vi "Sweep control.vi"(0 "Scan control":cluster{"Priority":u16, "Scan name":u16}[](array[cluster])=[{"Priority"=0, "Scan name"=1}, {"Priority"=1, "Scan name"=5}, {"Priority"=3, "Scan name"=0}, {"Priority"=2, "Scan name"=0}] {"Scan name" items=["OFF", "Vsg1", "Vsg2", "Vsgw", "Vbg", "Field", "Temp", "MW_freq", "MW_amplitude"]; "Priority" items=["Priority 0", "Priority 1", "Priority 2", "Priority 3", "Priority 4", "Priority 5"]}, 1 "Scan parameters":T2(array[cluster])=[{"DAQ Channel"=3, "Label"="\nappliedVsg=", "Scaled low"=-0.1, "Scaled high"=0.6, "Start"=-0.015, "End"=0.2, "Step"=0.001, "Scale?"=FALSE, "Output-Not Used"=0}, {"DAQ Channel"=3, "Label"="\nappliedField=", "Scaled low"=-0.175, "Scaled high"=0.775, "Start"=5.0, "End"=3.0, "Step"=0.1, "Scale?"=FALSE, "Output-Not Used"=2}, {"DAQ Channel"=3, "Label"="\nappliedVbg=", "Scaled low"=-0.11, "Scaled high"=0.31, "Start"=-1.55, "End"=3.0, "Step"=0.015, "Scale?"=FALSE, "Output-Not Used"=2}, {"DAQ Channel"=3, "Label"="\nappliedField=", "Scaled low"=-0.060000000000000005, "Scaled high"=0.14, "Start"=0.0, "End"=10000.0, "Step"=5000.0, "Scale?"=FALSE, "Output-Not Used"=2}] {"Step" format="%#_6p"; "End" format="%#_6p"; "Start" format="%#_6p"; "Scaled high" format="%#_6p"; "Scaled low" format="%#_6p"}, 3 "Comments":string="SA02703M.20141208\nVbg=0.25VV\n\nB= +0T\nSweep Vsg: -115mV to 200mV, 1mV steps\n\nlockin\n0: 1, current 2.5mV AC 400uV DC, 400mHz\n1: 2\n2: 3\n3: 5, \n4: 7, current\n5: 9, ", 4 "Experiment folder name":string="1 - seep Vsg") -> ()   [LabVIEW 2013]
uses:
  <userlib>/Levylab/DAQ-Lockin-SubVI/Lockin-4461_MultiChannel - IV 3.0 globals.vi
  Labview_Local/Lockin-4461_Multiple Inputs and Outputs_KH Folder/P/users1/Joe/Lockin-4461_3.0 4461-4462 Multichannel Folder/DAQ-Lockin-SubVI/Lock-in Globles Multiple Inputs and Outputs.vi
panel:
  in  "Channels: AO":T1={"AO amp (V)"=[0.002, 0.002, 0.002, 0.002, 0.002, 0.002, 0.002, 0.002], "AO DC (V)"=[0.0, 0.0, 0.0, 0.0, 0.0, 0.0, 0.0, 0.0], "AO f (Hz)"=[15.1, 15.11, 15.12, 15.13, 15.14, 15.15, 15.16, 15.17], "AO phi (deg)"=[0.0, 10.0, 20.0, 30.0, 40.0, 50.0, 60.0, 70.0], "function"=[enum."Sine Wave", enum."Sine Wave", enum."Sine Wave", enum."Sine Wave", enum."Sine Wave", enum."Sine Wave", enum."Sine Wave", enum."Sine Wave"]} {"AO DC (V)" format="%#_6p"; "AO amp (V)" format="%#_6p"}
  in  "Enum":enum16{"IV", "lockin", "IV/lockin continuous B"}(ring)
  in  "Additional action (indexing priority)":u16[](array[ring])=[4, 2, 4, 4] items=["Clear DAQ Tasks", "Check Temperature", "Check Field Value", "Wait", "Do Nothing"]
  in  "Number of IV curves":i32=1
  # "Instructions: \n1, you can put multiple scan names in one priority.\n2 OFF has to put in last priority"
  # "if you use the lockin\nprogram remember to\nset BG/SG parameters in\n'lockin_Vsg_multichannel.vi'"
  # "0"
  # "1"
  # "2"
  # "3"
  # "4"
  # "5"
  # "6"
  # "7"
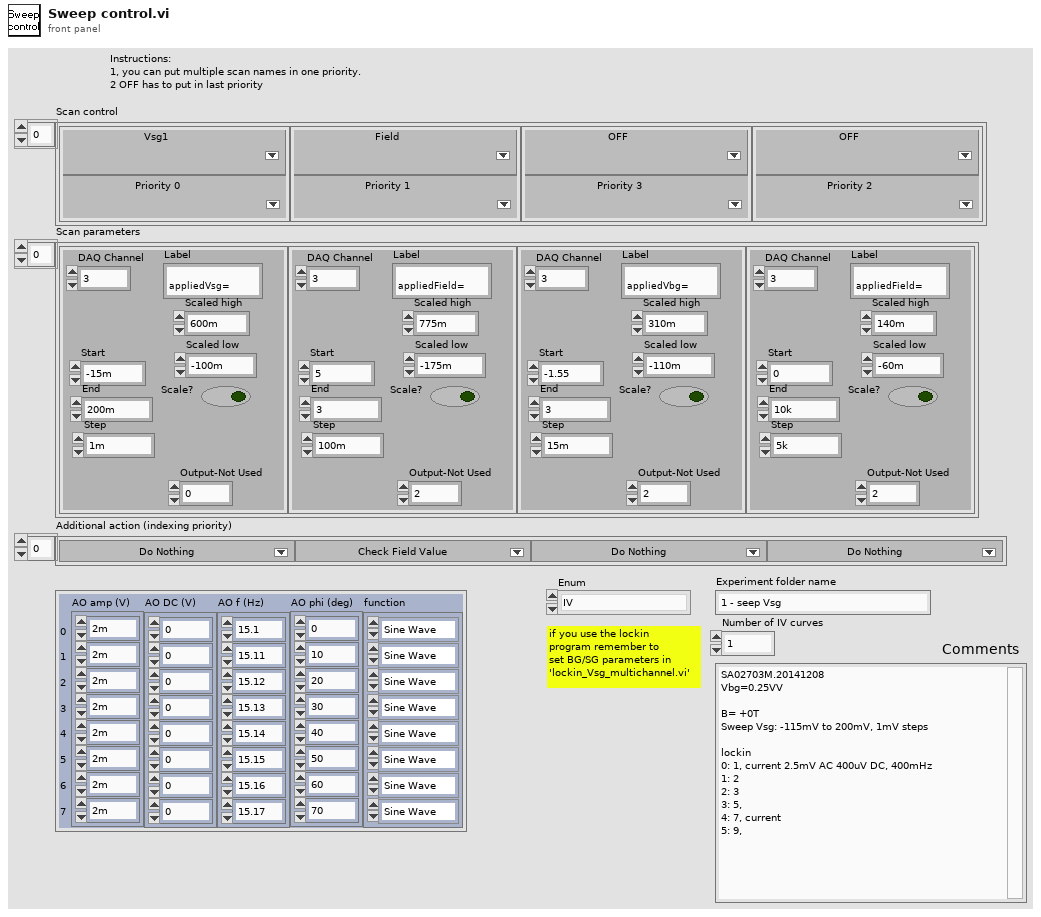
[diagram p1: front panel]
types:
  T1 = cluster{"AO amp (V)":dbl[], "AO DC (V)":dbl[], "AO f (Hz)":dbl[], "AO phi (deg)":dbl[], "function":enum16{"Sine Wave", "Triangle Wave", "Square Wave", "Sawtooth Wave"}[]}
  T2 = cluster{"DAQ Channel":i32, "Label":string, "Scaled low":dbl, "Scaled high":dbl, "Start":dbl, "End":dbl, "Step":dbl, "Scale?":bool, "Output-Not Used":i32}[]
  T3 = cluster{cluster{"DAQ Channel":i32, "Label":string, "Scaled low":dbl, "Scaled high":dbl, "Start":dbl, "End":dbl, "Step":dbl, "Scale?":bool}[]}[]
  T4 = cluster{cluster{"Priority":u16, "Scan name":u16}[]}[]
  T5 = cluster{cluster{"DAQ Channel":i32, "Label":string, "Scaled low":dbl, "Scaled high":dbl, "Start":dbl, "End":dbl, "Step":dbl, "Scale?":bool}[]}
  T6 = cluster{cluster{"Priority":u16, "Scan name":u16}[]}
  T7 = cluster{"DAQ Channel":i32, "Label":string, "Scaled low":dbl, "Scaled high":dbl, "Start":dbl, "End":dbl, "Step":dbl, "Scale?":bool}[]
  T8 = cluster{"Signal Type":enum16{"Sine Wave", "Triangle Wave", "Square Wave", "Sawtooth Wave"}, "DC":dbl, "Amplitude":dbl, "frequency":dbl, "Phase":dbl}[]
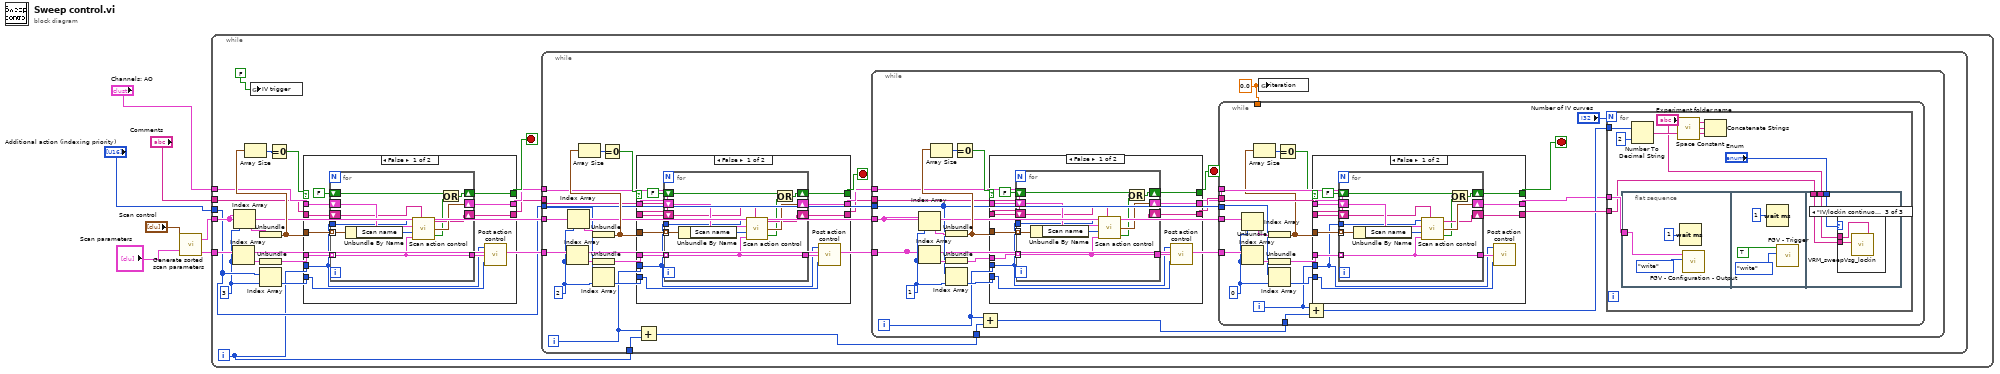
[diagram p0: block diagram]
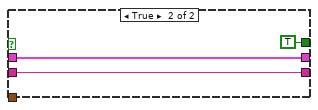
[diagram p2: hidden frame]
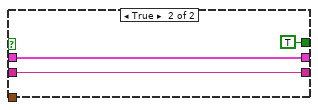
[diagram p3: hidden frame]
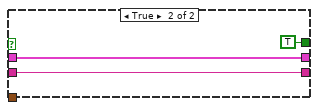
[diagram p4: hidden frame]
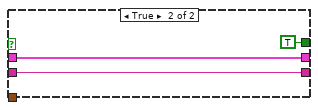
[diagram p5: hidden frame]
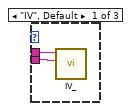
[diagram p6: hidden frame]
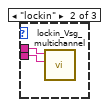
[diagram p7: hidden frame]
diagram:
  n1 = call <userlib>:"Generate sorted scan parameters.vi"("Scan parameters"="Scan parameters", "Scan control"="Scan control") -> ("Sorted scan parameters"=w2:T3, "Sorted scan control"=w4:T4)
  n2 = while {
    tunnel: "Comments" -> [w13]
    tunnel: "Channels: AO" -> [w14]
    tunnel: w2 -> [w20]
    tunnel: w4 -> [w19]
    tunnel: "Additional action (indexing priority)" -> [w15]
    i -> [w9]
    stop <- w17 stop-if-true
    w10 = 3
    n3 = Index Array(array=w20, index=w10) -> (element=w21:T5)
    n4 = Index Array(array=w19, index=w10) -> (element=w18:T6)
    n5 = global write "Lock-in Globles Multiple Inputs and Outputs.vi" "IV trigger"(FALSE) -> ()
    n6 = Unbundle(w18) -> (w23:cluster{"Priority":u16, "Scan name":u16}[])
    n7 = Array Size(array=w23) -> (size(s)=w24:i32)
    n8 = Unbundle(w21) -> (w22:T7)
    n9 = Index Array(array=w15, index=w10) -> (element=w16:u16)
    n10 = Equal To 0?(x=w24) -> (x = 0?=w25:bool)
    n11 = case shown="False" w25 {
      tunnel: w22 -> [w36 _]
      tunnel: [w35 w49] -> w12
      tunnel: [w34 w48] -> w11
      tunnel: [w28 TRUE ("Stop?")] -> w17
      tunnel: w23 -> [w33 _]
      tunnel: w9 -> [w30 _]
      tunnel: w16 -> [w31 _]
      tunnel: w14 -> [w27 w49]
      tunnel: w13 -> [w26 w48]
      frame False {
        n12 = for {
          tunnel: w33 -> [w47] mode=indexing
          tunnel: w36 -> [w40] mode=indexing
          tunnel: w30 -> [w41]
          shift-right: [w45] -> w35
          shift-left: w27 -> [w44]
          shift-right: [w43] -> w34
          shift-left: w26 -> [w42]
          tunnel: [w40] -> w32
          shift-right: [w37] -> w28
          shift-left: FALSE -> [w39]
          n13 = Unbundle By Name(w47) -> ("Scan name"=w46:u16)
          n14 = call <userlib>:"Scan action control.vi"("Index"=w41, "OSC Configuration"=w44, "Scan control"=w46, "Scan Parameters"=w40, "Comments"=w42) -> ("Comments out"=w43:string, "OSC Configuration out"=w45:T8, "Stop?"=w38:bool)
          n15 = Or(x=w39, y=w38) -> (x .or. y?=w37:bool)
        }
        n16 = call <userlib>:"Post action control.vi"("Action"=w31, "Scan Parameters"=w32, "Index"=w30) -> ()  [unwired: 1 out]
      }
      frame True {
      }
    }
    n17 = while {
      tunnel: w20 -> [w62]
      tunnel: w19 -> [w61]
      tunnel: w15 -> [w60]
      tunnel: w11 -> [w59]
      tunnel: w12 -> [w58]
      tunnel: w9 -> [w52]
      i -> [w53]
      stop <- w57 stop-if-true
      w54 = 2
      n18 = Index Array(array=w62, index=w54) -> (element=w68:T5)
      n19 = Index Array(array=w61, index=w54) -> (element=w69:T6)
      n20 = Unbundle(w69) -> (w66:cluster{"Priority":u16, "Scan name":u16}[])
      n21 = Array Size(array=w66) -> (size(s)=w64:i32)
      n22 = Unbundle(w68) -> (w67:T7)
      n23 = Index Array(array=w60, index=w54) -> (element=w65:u16)
      n24 = Equal To 0?(x=w64) -> (x = 0?=w63:bool)
      n25 = case shown="False" w63 {
        tunnel: w67 -> [w80 _]
        tunnel: w58 -> [w79 w94]
        tunnel: w59 -> [w78 w93]
        tunnel: [w77 w94] -> w56
        tunnel: [w76 w93] -> w55
        tunnel: [w70 TRUE ("Stop?")] -> w57
        tunnel: w66 -> [w75 _]
        tunnel: w53 -> [w72 _]
        tunnel: w65 -> [w73 _]
        frame False {
          n26 = for {
            tunnel: w75 -> [w91] mode=indexing
            tunnel: w80 -> [w84] mode=indexing
            tunnel: w72 -> [w85]
            shift-right: [w89] -> w77
            shift-left: w79 -> [w88]
            shift-right: [w87] -> w76
            shift-left: w78 -> [w86]
            tunnel: [w84] -> w74
            shift-right: [w81] -> w70
            shift-left: FALSE -> [w83]
            n27 = Unbundle By Name(w91) -> ("Scan name"=w90:u16)
            n28 = call <userlib>:"Scan action control.vi"("Index"=w85, "OSC Configuration"=w88, "Scan control"=w90, "Scan Parameters"=w84, "Comments"=w86) -> ("Comments out"=w87:string, "OSC Configuration out"=w89:T8, "Stop?"=w82:bool)
            n29 = Or(x=w83, y=w82) -> (x .or. y?=w81:bool)
          }
          n30 = call <userlib>:"Post action control.vi"("Action"=w73, "Scan Parameters"=w74, "Index"=w72) -> ()  [unwired: 1 out]
        }
        frame True {
        }
      }
      n31 = Add(x=w53, y=w52) -> (x+y=w51:i32)
      n32 = while {
        tunnel: w56 -> [w96]
        tunnel: w55 -> [w106]
        tunnel: w61 -> [w105]
        tunnel: w62 -> [w95]
        tunnel: w60 -> [w104]
        tunnel: w51 -> [w98]
        i -> [w99]
        stop <- w101 stop-if-true
        w100 = 1
        w114 = 0.0 ("iteration")
        n33 = Index Array(array=w105, index=w100) -> (element=w107:T6)
        n34 = Index Array(array=w95, index=w100) -> (element=w108:T5)
        n35 = Unbundle(w107) -> (w110:cluster{"Priority":u16, "Scan name":u16}[])
        n36 = Array Size(array=w110) -> (size(s)=w112:i32)
        n37 = Unbundle(w108) -> (w109:T7)
        n38 = Index Array(array=w104, index=w100) -> (element=w111:u16)
        n39 = Equal To 0?(x=w112) -> (x = 0?=w113:bool)
        n40 = Add(x=w99, y=w98) -> (x+y=w97:i32)
        n41 = case shown="False" w113 {
          tunnel: w109 -> [w125 _]
          tunnel: w96 -> [w124 w139]
          tunnel: w106 -> [w123 w138]
          tunnel: [w122 w139] -> w102
          tunnel: [w121 w138] -> w103
          tunnel: [w115 TRUE ("Stop?")] -> w101
          tunnel: w110 -> [w120 _]
          tunnel: w99 -> [w117 _]
          tunnel: w111 -> [w118 _]
          frame False {
            n42 = for {
              tunnel: w120 -> [w136] mode=indexing
              tunnel: w125 -> [w129] mode=indexing
              tunnel: w117 -> [w130]
              shift-right: [w134] -> w122
              shift-left: w124 -> [w133]
              shift-right: [w132] -> w121
              shift-left: w123 -> [w131]
              tunnel: [w129] -> w119
              shift-right: [w126] -> w115
              shift-left: FALSE -> [w128]
              n43 = Unbundle By Name(w136) -> ("Scan name"=w135:u16)
              n44 = call <userlib>:"Scan action control.vi"("Index"=w130, "OSC Configuration"=w133, "Scan control"=w135, "Scan Parameters"=w129, "Comments"=w131) -> ("Comments out"=w132:string, "OSC Configuration out"=w134:T8, "Stop?"=w127:bool)
              n45 = Or(x=w128, y=w127) -> (x .or. y?=w126:bool)
            }
            n46 = call <userlib>:"Post action control.vi"("Action"=w118, "Scan Parameters"=w119, "Index"=w117) -> ()  [unwired: 1 out]
          }
          frame True {
          }
        }
        n47 = while {
          tunnel: w105 -> [w158]
          tunnel: w95 -> [w157]
          tunnel: w102 -> [w153]
          tunnel: w103 -> [w152]
          tunnel: w104 -> [w148]
          tunnel: w114 -> [_]
          tunnel: w97 -> [w142]
          i -> [w143]
          stop <- w150 stop-if-true
          w145 = 0
          n48 = Index Array(array=w158, index=w145) -> (element=w156:T6)
          n49 = Index Array(array=w157, index=w145) -> (element=w155:T5)
          n50 = Unbundle(w156) -> (w149:cluster{"Priority":u16, "Scan name":u16}[])
          n51 = Array Size(array=w149) -> (size(s)=w147:i32)
          n52 = Unbundle(w155) -> (w154:T7)
          n53 = Index Array(array=w148, index=w145) -> (element=w144:u16)
          n54 = Equal To 0?(x=w147) -> (x = 0?=w146:bool)
          n55 = Add(x=w143, y=w142) -> (x+y=w141:i32)
          n56 = case shown="False" w146 {
            tunnel: w154 -> [w170 _]
            tunnel: w153 -> [w169 w184]
            tunnel: w152 -> [w168 w183]
            tunnel: [w167 w184] -> w140
            tunnel: [w166 w183] -> w151
            tunnel: [w161 TRUE ("Stop?")] -> w150
            tunnel: w149 -> [w165 _]
            tunnel: w143 -> [w160 _]
            tunnel: w144 -> [w163 _]
            frame False {
              n57 = for {
                tunnel: w165 -> [w181] mode=indexing
                tunnel: w170 -> [w174] mode=indexing
                tunnel: w160 -> [w175]
                shift-right: [w179] -> w167
                shift-left: w169 -> [w178]
                shift-right: [w177] -> w166
                shift-left: w168 -> [w176]
                tunnel: [w174] -> w164
                shift-right: [w171] -> w161
                shift-left: FALSE -> [w173]
                n58 = Unbundle By Name(w181) -> ("Scan name"=w180:u16)
                n59 = call <userlib>:"Scan action control.vi"("Index"=w175, "OSC Configuration"=w178, "Scan control"=w180, "Scan Parameters"=w174, "Comments"=w176) -> ("Comments out"=w177:string, "OSC Configuration out"=w179:T8, "Stop?"=w172:bool)
                n60 = Or(x=w173, y=w172) -> (x .or. y?=w171:bool)
              }
              n61 = call <userlib>:"Post action control.vi"("Action"=w163, "Scan Parameters"=w164, "Index"=w160) -> ()  [unwired: 1 out]
            }
            frame True {
            }
          }
          n62 = for {
            N: "Number of IV curves" -> [_]
            tunnel: w140 -> [w192]
            tunnel: w151 -> [w186]
            tunnel: w141 -> [w190]
            n63 = flat-sequence {
              tunnel: w192 -> [w194]
              tunnel: "Enum" -> [w201]
              tunnel: w186 -> [w200]
              tunnel: "Experiment folder name" -> [w199]
              frame #0 {
                n64 = Wait (ms)(milliseconds to wait=u32 1) -> ()  [unwired: 1 out]
                n65 = call "FGV - Configuration - Output.vi"("Function"=enum16{"write", "read"}."write", "Channels: AO"=w194) -> ()  [unwired: 4 in, 2 out]
              }
              frame #1 {
                n66 = Wait (ms)(milliseconds to wait=u32 1) -> ()  [unwired: 1 out]
                n67 = call "FGV - Trigger.vi"("Function"=enum16{"write", "read"}."write", "Trigger"=TRUE) -> ()  [unwired: 4 in, 2 out]
              }
              frame #2 {
                n68 = case shown="\"IV/lockin continuous B\"" w201 {
                  tunnel: w200 -> [w203 w204 w206]
                  tunnel: w199 -> [w202 w205 w207]
                  frame "IV", Default {
                    n69 = call "IV_.vi"("Notes"=w203, "Experiment folder name"=w202) -> ()  [unwired: 10 in]
                  }
                  frame "lockin" {
                    n70 = call "lockin_Vsg_multichannel.vi"("Comments"=w204, "ITX folder"=w205) -> ()  [unwired: 10 in]
                  }
                  frame "IV/lockin continuous B" {
                    n71 = call "VRM_sweepVsg_lockin.vi"("Comments"=w206, "ITX folder"=w207) -> ()  [unwired: 7 in, 1 out]
                  }
                }
              }
            }
            n72 = Number To Decimal String(number=w190, width (-)=i16 2) -> (decimal integer string=w189:string)
            n73 = call <vilib>:"Space Constant.vi"() -> ("String"=w188:string)
            n74 = Concatenate Strings("Experiment folder name", w188, w189) -> ()  [unwired: 1 out]
          }
        }
        n75 = global write "Lockin-4461_MultiChannel - IV 3.0 globals.vi" "iteration"(w114) -> ()
      }
    }
  }
